vi "Get Type.vi"(11 "String in":refnum<class "String.lvclass">) -> (3 "Type":string)   [LabVIEW 2019, in "String.lvclass"]
uses:
  <vilib>/gpm_packages/@cs/data-type-serializer/source/String/String.lvclass
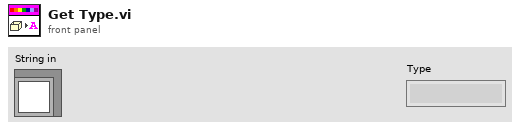
[diagram p1: front panel]
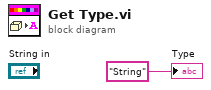
[diagram p0: block diagram]
diagram:
  "Type" <- "String" ("Type")
